vi "Instrument.Temperhum.GetPublicEvents.vi"(8 "error in (no error)":errorcluster, 11 "Instrument.Temperhum in":refnum<class "Instrument.Temperhum.lvclass">) -> (0 "error out":errorcluster, 2 "Temperhum Public Events":T1, 3 "Instrument.Temperhum out":refnum<class "Instrument.Temperhum.lvclass">)   [LabVIEW 2019, in "Instrument.Temperhum.lvclass"]
uses:
  Instrument.Temperhum.lvclass
  Typedefs/PublicEvents--Cluster.ctl
  Typedefs/PublicEvents--Instrument.Temperhum.Get PGSQL Info.ctl
  Instrument.Temperhum.lvclass/Instrument.Temperhum.ctl
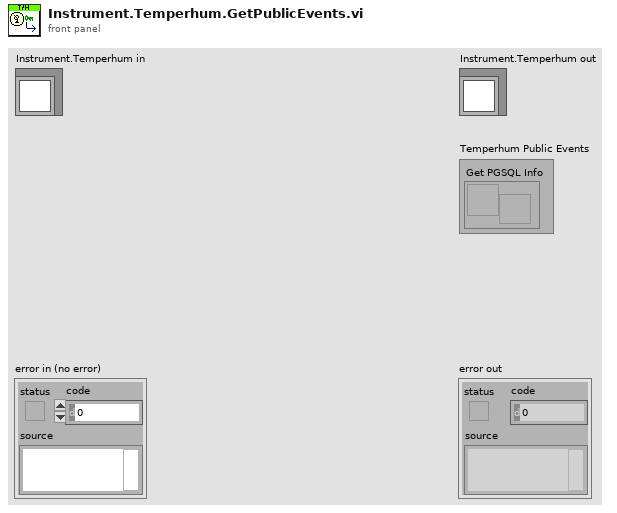
[diagram p1: front panel]
types:
  T1 = typedef "Instrument.Temperhum.lvclass/PublicEvents--Cluster.ctl" = cluster{"Get PGSQL Info":refnum<user-event>}
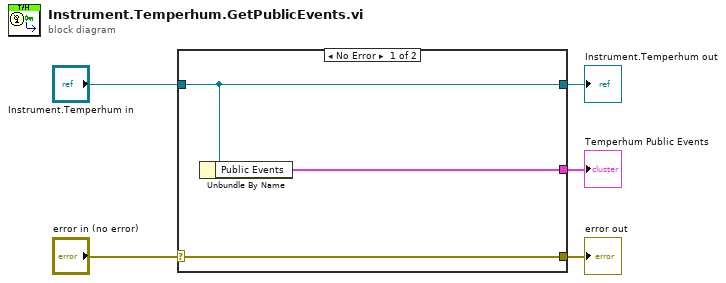
[diagram p0: block diagram]
diagram:
  n1 = case shown="No Error" "error in (no error)" {
    selector: "error in (no error)" -> [w8 w9]
    tunnel: [w8 w9] -> w4
    tunnel: [w7 w10] -> w2
    tunnel: "Instrument.Temperhum in" -> [w7 w10]
    tunnel: [w6 _] -> w1
    frame No Error {
      n2 = Unbundle By Name(w7) -> ("Public Events"=w6:T1)
    }
    frame Error {
    }
  }
  "error out" <- w4
  "Instrument.Temperhum out" <- w2
  "Temperhum Public Events" <- w1
